vi "TurnDegrees to MM Setpoints.vi"(2 "Turn Degrees":dbl) -> (0 "Right MM SetpointFT":dbl, 1 "Left MM SetpointFT":dbl)   [LabVIEW 2018]
panel:
  in  "Track Width(ft)":dbl=1.7
  # "Will Need to create some \nnumbers for trig in constants.vi\nFor example: Trackwidth\n\n\n\n\n\n\n\n\n\n\n\n\n\n\n\n\n\nProduct of Cyril Ng and Hermela Benyam"
  # "POSITIVE IS CLOCKWISE ACCORDING TO THIS"
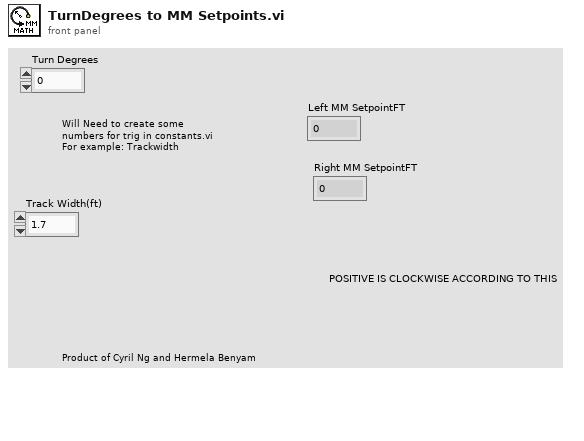
[diagram p1: front panel]
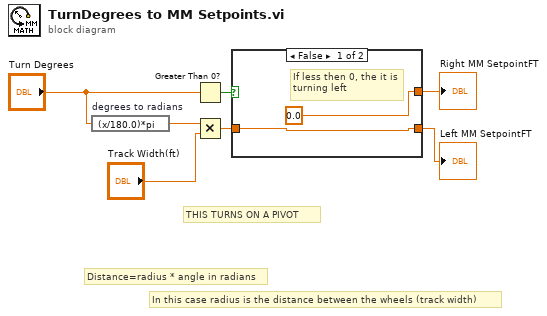
[diagram p0: block diagram]
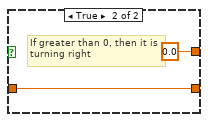
[diagram p2: hidden frame]
diagram:
  # "In this case radius is the distance between the wheels (track width)"
  # "THIS TURNS ON A PIVOT"
  # "Distance=radius * angle in radians"
  n1 = expression code="(x/180.0)*pi" "degrees to radians"("Turn Degrees") -> (w2:dbl)
  n2 = Greater Than 0?(x="Turn Degrees") -> (x > 0?=w5:bool)
  n3 = Multiply(x=w2, y="Track Width(ft)") -> (x*y=w3:dbl)
  n4 = case shown="False" w5 {
    tunnel: w3 -> [w8 w10]
    tunnel: [0.0 0.0] -> w6
    tunnel: [w8 w10] -> w7
    frame False {
      # "If less then 0, the it is\nturning left"
    }
    frame True {
      # "If greater than 0, then it is\nturning right"
    }
  }
  "Right MM SetpointFT" <- w6
  "Left MM SetpointFT" <- w7
